vi "Setup subWorker - DataSave.vi"(8 "error in":errorcluster, 11 "DataAcquire Worker in":refnum<class "DataAcquire Worker.lvclass">) -> (0 "error out":errorcluster, 3 "DataAcquire Worker out":refnum<class "DataAcquire Worker.lvclass">)   [LabVIEW 2018, in "DataAcquire Worker.lvclass"]
doc: "<b>Note: Do not change the code in this VI!</b>\nThis VI performs a setup of all the statically-linked subWorkers that belong to the Worker that calls this VI. This VI is created automatically by the 'Create/Add Worker' tool and must be called <b>before</b> any statically linked subWorkers are called."
uses:
  DataAcquire Worker.lvclass
  DataAcquire Worker.lvclass/DataAcquire Worker.ctl
  DataSave Worker/DataSave Worker.lvclass
  D:/Program Files (x86)/National Instruments/LabVIEW 2018/vi.lib/addons/_Workers/Library/Classes/Worker/Worker.lvclass
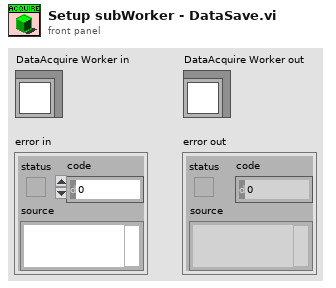
[diagram p1: front panel]
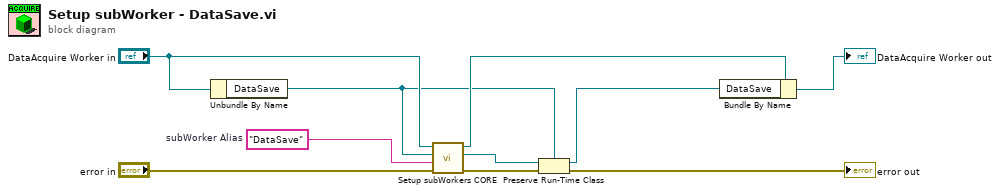
[diagram p0: block diagram]
diagram:
  w6 = "DataSave"  # subWorker Alias
  n1 = Unbundle By Name("DataAcquire Worker in") -> ("DataSave"=w3:refnum<class "DataSave Worker.lvclass">)
  n2 = call-dynamic "Setup subWorkers CORE.vi"("error in"="error in", "subWorker Alias"=w6, "subWorker"=w3, "Worker"="DataAcquire Worker in") -> ("error out"=w5:errorcluster, "subWorker out"=w1:refnum<class "Worker.lvclass">, "Worker out"=w8:refnum<class "DataAcquire Worker.lvclass">)  [unwired: 5 in]
  n3 = Preserve Run-Time Class(object in=w1, error in=w5, 2:w3) -> (object out=w2:refnum<class "DataSave Worker.lvclass">, error out=→"error out":errorcluster)
  n4 = Bundle By Name(cluster=w8, "DataSave"=w2) -> (→"DataAcquire Worker out":refnum<class "DataAcquire Worker.lvclass">)
